vi "read_data.vi"(8 "error in (no error)":errorcluster, 11 "Naive_bayes in":refnum<class "Naive_bayes.lvclass">) -> (0 "error out":errorcluster, 2 "data":T1, 3 "Naive_bayes out":refnum<class "Naive_bayes.lvclass">)   [LabVIEW 2020, in "Naive_bayes.lvclass"]
uses:
  Naive_bayes.lvclass
  Controls/naive_bayes_data.ctl
  Naive_bayes.lvclass/Naive_bayes.ctl
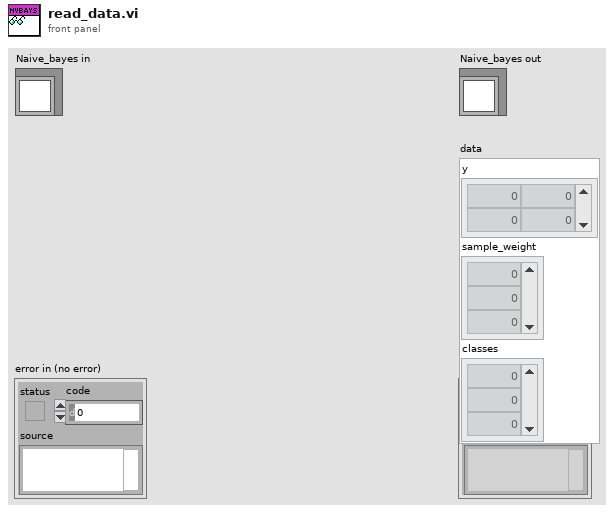
[diagram p1: front panel]
types:
  T1 = typedef "naive_bayes_data.ctl" = cluster{"y":dbl[][], "sample_weight":dbl[], "classes":dbl[]}
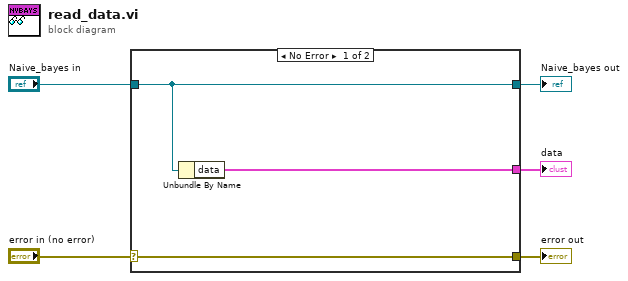
[diagram p0: block diagram]
diagram:
  n1 = case shown="No Error" "error in (no error)" {
    selector: "error in (no error)" -> [w8 w9]
    tunnel: [w8 w9] -> w4
    tunnel: [w7 w10] -> w2
    tunnel: "Naive_bayes in" -> [w7 w10]
    tunnel: [w6 _] -> w1
    frame No Error {
      n2 = Unbundle By Name(w7) -> ("data"=w6:T1)
    }
    frame Error {
    }
  }
  "error out" <- w4
  "Naive_bayes out" <- w2
  "data" <- w1
